vi "mxwScript_Cmnd2Str_runAddOn.vi"(8 "error in (no error)":errorcluster, 11 "data":variant) -> (0 "error out":errorcluster, 3 "outputString":string)   [LabVIEW 2020]
uses:
  codeGenAPISupport.llb/cgAPI_mxwScript_RunAddOnInfo.ctl
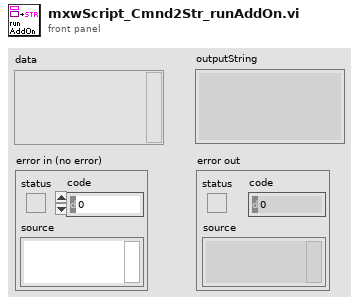
[diagram p1: front panel]
types:
  T1 = typedef "cgAPI_mxwScript_RunAddOnInfo.ctl" = cluster{"context":string, "viPath":path, "parameters":cluster{"label":string, "value":variant}[]}
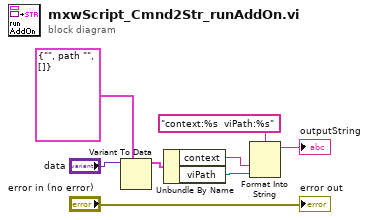
[diagram p0: block diagram]
diagram:
  n1 = Variant To Data(type=T1 {"context"="", "viPath"=path "", "parameters"=[]} ("RunAddOn info"), Variant="data") -> (data=w5:T1)  [unwired: 1 in, 1 out]
  n2 = Unbundle By Name(w5) -> ("context"=w2:string, "viPath"=w3:path)
  n3 = Format Into String(format string="context:%s  viPath:%s", w2, w3) -> (resulting string=→"outputString":string)  [unwired: 2 in, 1 out]
  "error out" <- "error in (no error)"
